vi "Edgertronic_OpenQTPlayer.vi"(3 "Path":path=path "/Volumes/Kim/Users/crogers/Dropbox (Rogers)/LVPresent/Talk/Movies/DrEs/Bacon Thrower.mp4") -> ()   [LabVIEW 2015]
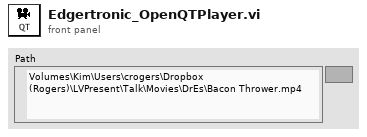
[diagram p1: front panel]
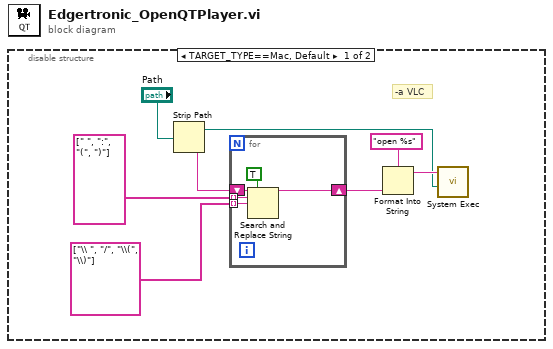
[diagram p0: block diagram]
diagram:
  n1 = disable-structure shown="TARGET_TYPE==Mac, Default" {
    frame condition #0 (active) {
      # "-a VLC"
      n2 = Strip Path(path="Path") -> (stripped path=w2:path, name=w3:string)
      n3 = for {
        shift-right: [w11] -> w6
        shift-left: w3 -> [w13]
        tunnel: string[] [" ", ":", "(", ")"] -> [w10] mode=indexing
        tunnel: string[] ["\\ ", "/", "\\(", "\\)"] -> [w9] mode=indexing
        n4 = Search and Replace String(replace all?=TRUE ("replace all? (F)"), input string=w13, search string=w10, replace string=w9) -> (result string=w11:string)  [unwired: 4 in, 3 out]
      }
      n5 = Format Into String(format string="open %s", w6) -> (resulting string=w4:string)  [unwired: 2 in, 1 out]
      n6 = call <vilib>:"System Exec.vi"("working directory"=w2, "command line"=w4) -> ()  [unwired: 6 in, 4 out]
    }
    frame condition #1 {
    }
  }
